vi "configureAcquisition.vi"(8 "error in (no error)":errorcluster, 11 "AndorIKonAcquisitor in":refnum<class "AndorIKonAcquisitor.lvclass">) -> (0 "error out":errorcluster, 3 "AndorIKonAcquisitor out":refnum<class "AndorIKonAcquisitor.lvclass">)   [LabVIEW 2011, in "Hardware.lvlib" / "Channels.lvlib" / "AndorIKonAcquisitor.lvclass"]
uses:
  AndorIKonAcquisitor.lvclass
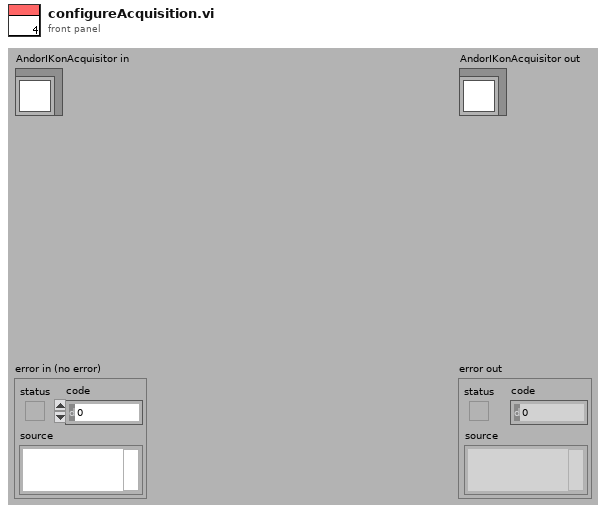
[diagram p1: front panel]
types:
  T1 = cluster{"Acquisition mode":dbl, "Readout Mode":dbl, "Gain":dbl}
  T2 = cluster{"Vertical Binning":dbl, "Horizontal Binning":dbl, "SubArea Height":dbl, "SubAreaWidth":dbl, "Offset":dbl, "Number of Tracks":dbl, "Track Positions":cluster{"Top":dbl, "Bottom ":dbl}[], "subArea Coordinate":dbl[]}
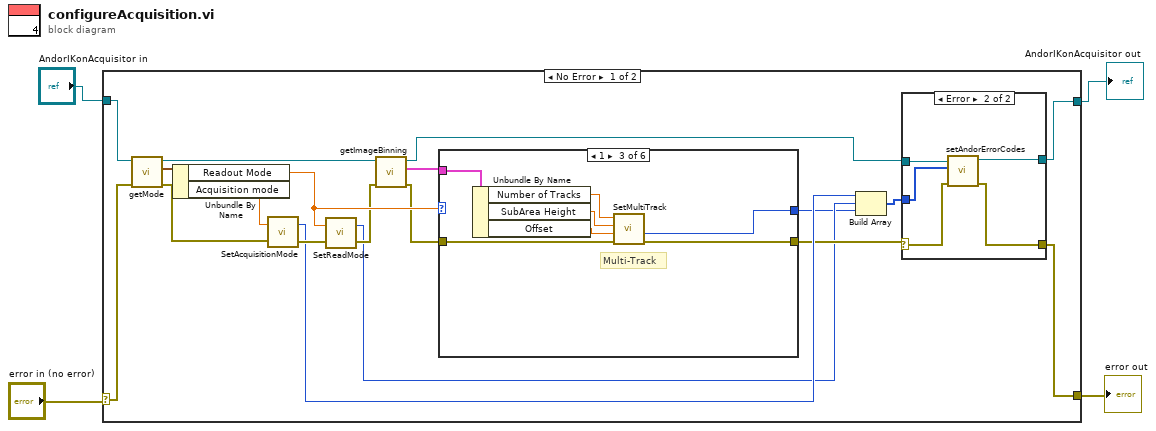
[diagram p0: block diagram]
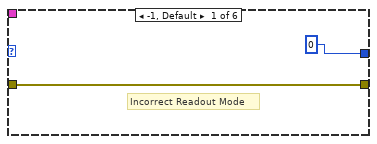
[diagram p2: hidden frame]
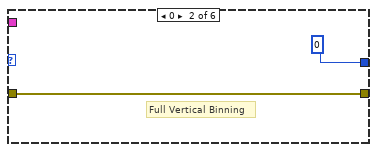
[diagram p3: hidden frame]
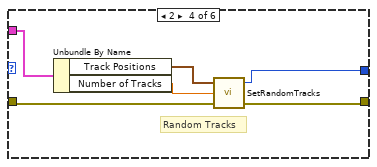
[diagram p4: hidden frame]
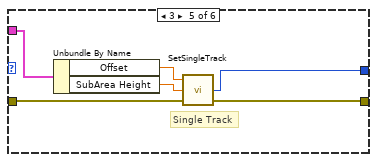
[diagram p5: hidden frame]
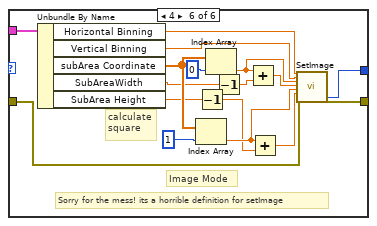
[diagram p6: hidden frame]
diagram:
  n1 = case shown="No Error" "error in (no error)" {
    selector: "error in (no error)" -> [w22 w71]
    tunnel: "AndorIKonAcquisitor in" -> [w18 w72]
    tunnel: [w16 w72] -> w2
    tunnel: [w17 w71] -> w1
    frame No Error {
      n2 = call-dynamic "getMode.vi"("error in (no error)"=w22, "CameraAcquisitor.lvclass in"=w18) -> ("error out"=w20:errorcluster, "Mode"=w21:T1, "CameraAcquisitor.lvclass out"=w11:refnum<class "AndorIKonAcquisitor.lvclass">)  [unwired: 7 in]
      n3 = Unbundle By Name(w21) -> ("Readout Mode"=w13:dbl, "Acquisition mode"=w19:dbl)
      n4 = call <userlib>:"SetAcquisitionMode.vi"("error in (no error)"=w20, "mode"=w19) -> ("error out"=w23:errorcluster, "DLL error code"=w15:u32)
      n5 = call <userlib>:"SetReadMode.vi"("error in (no error)"=w23, "mode"=w13) -> ("error out"=w9:errorcluster, "DLL error code"=w6:u32)
      n6 = call-dynamic "getImageBinning.vi"("error in (no error)"=w9, "CameraAcquisitor.lvclass in"=w11) -> ("error out"=w8:errorcluster, "Image Binning"=w7:T2, "CameraAcquisitor.lvclass out"=w10:refnum<class "AndorIKonAcquisitor.lvclass">)  [unwired: 7 in]
      n7 = case shown="1" w13 {
        tunnel: [0 0 w32 w38 w44 w51] -> w5
        tunnel: [w25 w26 w33 w39 w45 w52] -> w12
        tunnel: w8 -> [w25 w26 w34 w40 w46 w63]
        tunnel: w7 -> [_ _ w31 w37 w43 w62]
        frame -1, Default {
          # "Incorrect Readout Mode"
        }
        frame 0 {
          # "Full Vertical Binning"
        }
        frame 1 {
          # "Multi-Track"
          n8 = Unbundle By Name(w31) -> ("Number of Tracks"=w30:dbl, "SubArea Height"=w29:dbl, "Offset"=w28:dbl)
          n9 = call <userlib>:"SetMultiTrack.vi"("error in (no error)"=w34, "offset"=w28, "height"=w29, "number"=w30) -> ("error out"=w33:errorcluster, "DLL error code"=w32:u32)  [unwired: 2 out]
        }
        frame 2 {
          # "Random Tracks"
          n10 = Unbundle By Name(w37) -> ("Track Positions"=w35:cluster{"Top":dbl, "Bottom ":dbl}[], "Number of Tracks"=w36:dbl)
          n11 = call <userlib>:"SetRandomTracks.vi"("error in (no error)"=w40, "# of Tracks"=w36, "tracks"=w35) -> ("error out"=w39:errorcluster, "DLL error code"=w38:u32)  [unwired: 1 in]
        }
        frame 3 {
          # "Single Track"
          n12 = Unbundle By Name(w43) -> ("Offset"=w42:dbl, "SubArea Height"=w41:dbl)
          n13 = call <userlib>:"SetSingleTrack.vi"("error in (no error)"=w46, "height"=w41, "centre"=w42) -> ("error out"=w45:errorcluster, "DLL error code"=w44:u32)  [unwired: 1 in]
        }
        frame 4 {
          # "calculate\nsquare"
          # "Sorry for the mess! its a horrible definition for setImage"
          # "Image Mode"
          n14 = Unbundle By Name(w62) -> ("Horizontal Binning"=w50:dbl, "Vertical Binning"=w49:dbl, "subArea Coordinate"=w58:dbl[], "SubAreaWidth"=w55:dbl, "SubArea Height"=w56:dbl)
          n15 = Index Array(array=w58, index=1) -> (element=w54:dbl)
          n16 = Decrement(x=w56) -> (x-1=w48:dbl)
          n17 = Index Array(array=w58, index=0) -> (element=w60:dbl)
          n18 = Decrement(x=w55) -> (x-1=w47:dbl)
          n19 = Add(x=w60, y=w47) -> (x+y=w59:dbl)
          n20 = Add(x=w54, y=w48) -> (x+y=w53:dbl)
          n21 = call <userlib>:"SetImage.vi"("hbin"=w50, "vbin"=w49, "hstart"=w60, "hend"=w59, "vstart"=w54, "vend"=w53, "error in (no error)"=w63) -> ("DLL error code"=w51:u32, "error out"=w52:errorcluster)  [unwired: 19 in]
        }
      }
      n22 = Build Array(w15, w6, w5) -> (w14:u32[])
      n23 = case shown="Error" w12 {
        selector: w12 -> [w65 w70]
        tunnel: w10 -> [w64 w66]
        tunnel: [w64 w68] -> w16
        tunnel: [w65 w69] -> w17
        tunnel: w14 -> [_ w67]
        frame No Error {
        }
        frame Error {
          n24 = call-dynamic "setAndorErrorCodes.vi"("error in (no error)"=w70, "Andor Error Codes"=w67, "AndorIKonAcquisitor.lvclass in"=w66) -> ("error out"=w69:errorcluster, "AndorIKonAcquisitor.lvclass out"=w68:refnum<class "AndorIKonAcquisitor.lvclass">)  [unwired: 7 in]
        }
      }
    }
    frame Error {
    }
  }
  "error out" <- w1
  "AndorIKonAcquisitor out" <- w2
